vi "Create CIPC_DAQ_FIFO Config.vi"(11 "DAQ FIFO Config":T1={"Max Samples"=100000, "Max Channels"=8, "FIFO Flags"={"Backpressure"=FALSE}}) -> (3 "Flattened FIFO Config":u8[](array[numeric]))   [LabVIEW 2021, in "ChannelCommon.lvlib"]
doc: "This will create the flattened FIFO configuration used to override the default settings when creating a new FIFO reader or writer. If no configuration is provided the default for that FIFO type will be used. \n\nThis configuration is also used on tag writers with variable length input such as string tags. For tags only the Max Bytes/Msg element is used and other fields are ignored. \n\nIf additional custom data is needed by the FIFO type this can be appended to the end of the flattened data. This custom data will be FIFO specific and is not commonly used."
uses:
  ChannelCommon.lvlib
  typedef/New CIPC_DAQ_FIFO Config.ctl
  typedef/FIFO Flags.ctl
  typedef/FIFO Config.ctl
  <vilib>/CIF Foundation/CIF Utilities/DataTypes/Flatten Unflatten/Flatten U64.vi
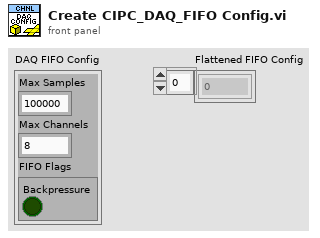
[diagram p1: front panel]
types:
  T1 = typedef "ChannelCommon.lvlib/New CIPC_DAQ_FIFO Config.ctl" = cluster{"Max Samples":u64, "Max Channels":u64, "FIFO Flags":T2}
  T2 = typedef "ChannelCommon.lvlib/FIFO Flags.ctl" = cluster{"Backpressure":bool}
  T3 = typedef "ChannelCommon.lvlib/FIFO Config.ctl" = cluster{"Max Bytes/Msg":u64, "Max Msg/FIFO":u64, "Flags":u64, "Custom Data":u8[]}
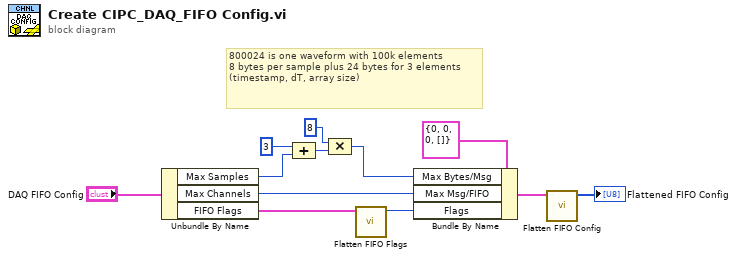
[diagram p0: block diagram]
diagram:
  # "800024 is one waveform with 100k elements\n8 bytes per sample plus 24 bytes for 3 elements (timestamp, dT, array size)"
  n1 = Unbundle By Name("DAQ FIFO Config") -> ("Max Samples"=w5:u64, "Max Channels"=w9:u64, "FIFO Flags"=w11:T2)
  n2 = Compound Arithmetic op=ADD(u64 3 ("value"), w5) -> (w4:u64)
  n3 = Compound Arithmetic op=MULTIPLY(u64 8 ("value"), w4) -> (w1:u64)
  n4 = call "Flatten FIFO Flags.vi"("Flags"=w11) -> ("FIFO Flags"=w10:u64)  [unwired: 10 in]
  n5 = Bundle By Name(cluster=T3 {"Max Bytes/Msg"=0, "Max Msg/FIFO"=0, "Flags"=0, "Custom Data"=[]} ("FIFO Config in"), "Max Bytes/Msg"=w1, "Max Msg/FIFO"=w9, "Flags"=w10) -> (w8:T3)
  n6 = call "Flatten FIFO Config.vi"("FIFO Config in"=w8) -> ("Flattened FIFO Config"=→"Flattened FIFO Config":u8[])  [unwired: 10 in]
